vi "Update_protocol_definition_values.vi"(5 "index (col)":i32, 7 "index (row)":i32, 8 "error in":errorcluster, 9 "Protocol name":string, 10 "Value":dbl, 11 "Protocol definition ref":refnum<vi>) -> (0 "error out":errorcluster)   [LabVIEW 2013]
panel:
  in  "MODBUS Register":i32
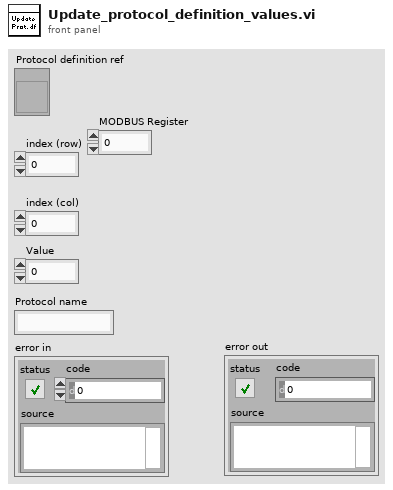
[diagram p1: front panel]
types:
  T1 = cluster{"Variables":u16, "Value":dbl, "Error":bool, "Input":u16, "time stamp":timestamp, "Protocol name":string}[][]
  T2 = cluster{"Variables":u16, "Value":dbl, "Error":bool, "Input":u16, "time stamp":timestamp, "Protocol name":string}
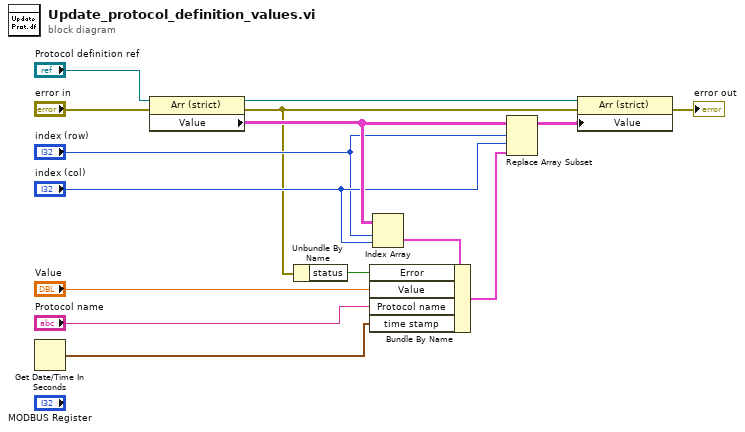
[diagram p0: block diagram]
diagram:
  n1 = Get Date/Time In Seconds() -> (seconds since 1Jan1904=w1:timestamp)
  n2 = property class="Arr (strict)"(reference="Protocol definition ref", error in="error in") -> (reference out=w14:refnum<vi>, error out=w4:errorcluster, "Value"=w15:T1)
  n3 = Unbundle By Name(w4) -> ("status"=w2:bool)
  n4 = Index Array(array=w15, index (row)="index (row)", index (col)="index (col)") -> (element=w11:T2)
  n5 = Bundle By Name(cluster=w11, "Error"=w2, "Value"="Value", "Protocol name"="Protocol name", "time stamp"=w1) -> (w12:T2)
  n6 = Replace Array Subset(array=w15, new element=w12, index (row)="index (row)", index (col)="index (col)") -> (w13:T1)
  n7 = property class="Arr (strict)"(reference=w14, error in=w4, "Value"=w13) -> (error out=→"error out":errorcluster)  [unwired: 1 out]
